vi "Test 2.vi"() -> ()   [LabVIEW 2019]
panel:
  out "TCP Connected":bool
  out "Acknowladged":bool
  in  "Beam":bool
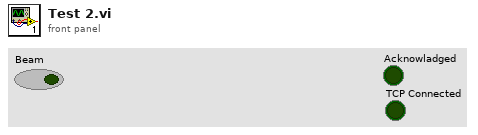
[diagram p1: front panel]
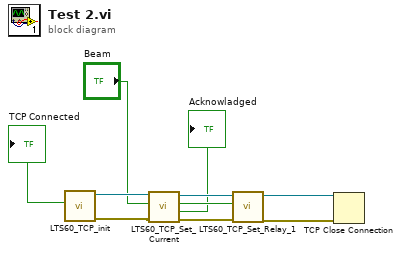
[diagram p0: block diagram]
diagram:
  n1 = call "LTS60_TCP_init.vi"() -> ("error out"=w3:errorcluster, "TCP Connected"=→"TCP Connected":bool, "connection ID out"=w7:refnum<k5>)  [unwired: 9 in]
  n2 = call "LTS60_TCP_Set_Current.vi"("error in (no error)"=w3, "Beam"="Beam", "connection ID"=w7) -> ("error out"=w9:errorcluster, "Acknowladged"=→"Acknowladged":bool, "Beam out"=w8:bool, "connection ID out"=w10:refnum<k5>)  [unwired: 5 in]
  n3 = call "LTS60_TCP_Set_Relay_1.vi"("error in (no error)"=w9, "Beam"=w8, "connection ID"=w10) -> ("error out"=w5:errorcluster, "connection ID out"=w4:refnum<k5>)  [unwired: 5 in, 2 out]
  n4 = TCP Close Connection(connection ID=w4, error in (no error)=w5) -> ()  [unwired: 1 in, 2 out]
